vi "Sequencer Main.vi"() -> ()   [LabVIEW 2018] (continued)
                                n1754 = in-place {
                                in-place-border: [w3148] -> w3129
                                in-place-border: w3133 -> [w3147]
                                n1755 = global read "Global Variable.vi" "Rd PID"() -> (w3149:string)
                                n1756 = Equal?(x=w3149, y=w3147) -> (x = y?=w3148:bool)
                                n1757 = global write "Global Variable.vi" "Rd PID RFID"(w3147) -> ()
                                }
                                n1758 = case shown="False" w3129 {
                                tunnel: [w3141 w3142] -> w3131
                                tunnel: w3130 -> [w3140 w3142]
                                frame False {
                                n1759 = Concatenate Strings(w3140, " (False)" ("string")) -> (w3141:string)
                                }
                                frame True {
                                }
                                }
                                n1760 = in-place {
                                in-place-border: w3132 -> [w3144]
                                in-place-border: w3137 -> [w3146]
                                in-place-border: w3138 -> [w3145]
                                in-place-border: [w3143] -> w3135
                                n1761 = In Range and Coerce(upper limit=w3146, x=w3144, lower limit=w3145) -> (In Range?=w3143:bool)  [unwired: 1 out]
                                }
                                n1762 = And(x=w3135, y=w3129) -> (x .and. y?=w3136:bool)
                              }
                            }
                          }
                          n1763 = local read "Debugging"() -> (w3066:bool)
                          n1764 = global read "Global Variable.vi" "Retest Cnt"() -> (w3068:i16)
                          n1765 = in-place {
                            in-place-border: w3070 -> [w3099]
                            in-place-border: [w3098] -> w3069
                            in-place-border: [w3097] -> w3064
                            in-place-border: [w3096] -> w3063
                            # "GoTo Test-nmb"
                            # "ReTest Cyckles"
                            n1766 = Index Array(array=w3099, index #1=0 ("index"), index #2=1 ("index"), index #3=2 ("index")) -> (element #1=w3102:string, element #2=w3101:string, element #3=w3100:string)
                            n1767 = Decimal String To Number(string=w3100) -> (number=w3097:i32)  [unwired: 2 in, 1 out]
                            n1768 = Decimal String To Number(string=w3101) -> (number=w3096:i32)  [unwired: 2 in, 1 out]
                            n1769 = To Upper Case(1:w3102) -> (0:w3098:string)
                          }
                          n1770 = case shown="True" w3074 {
                            tunnel: [enum16{"Idle", "PASS", "FALSE"}."FALSE" ("Step Test Result") enum16{"Idle", "PASS", "FALSE"}."PASS" ("Step Test Result")] -> w3079
                            frame False {
                            }
                            frame True {
                            }
                          }
                          n1771 = Equal?(x=w3068, y=i16 0) -> (x = y?=w3065:bool)
                          n1772 = case shown="False" w3066 {
                            tunnel: w3069 -> [w3083 _]
                            tunnel: w3065 -> [w3080 _]
                            tunnel: w3064 -> [w3082 _]
                            tunnel: w3063 -> [w3081 _]
                            frame False {
                              n1773 = case shown="\"FALSE\"" w3083 {
                                tunnel: w3080 -> [_ w3084]
                                tunnel: w3082 -> [_ w3086]
                                tunnel: w3081 -> [_ w3085]
                                frame "Idle", Default {
                                }
                                frame "FALSE" {
                                n1774 = case shown="False" w3084 {
                                tunnel: w3086 -> [_ w3093]
                                tunnel: w3085 -> [w3088 w3095]
                                frame False {
                                n1775 = global read "Global Variable.vi" "Retest Cnt"() -> (w3091:i16)
                                n1776 = global write "Global Variable.vi" "Retest Step Nmb"(w3088) -> ()
                                n1777 = global write "Global Variable.vi" "Retest ON"(TRUE ("Retest ON")) -> ()
                                n1778 = Decrement(x=w3091) -> (x-1=w3090:i16)
                                n1779 = global write "Global Variable.vi" "Retest Cnt"(w3090) -> ()
                                n1780 = Wait (ms)(milliseconds to wait=u32 1000) -> ()  [unwired: 1 out]
                                }
                                frame True {
                                # "if(Retest-OFF & Cnt=0)"
                                n1781 = Decrement(x=w3093) -> (x-1=w3092:i32)
                                n1782 = global write "Global Variable.vi" "Retest Step Nmb"(w3095) -> ()
                                n1783 = global write "Global Variable.vi" "Retest ON"(TRUE ("Retest ON")) -> ()
                                n1784 = global write "Global Variable.vi" "Retest Cnt"(w3092) -> ()
                                }
                                }
                                }
                              }
                            }
                            frame True {
                            }
                          }
                        }
                        frame 46 {
                          # "GoTo Test-nmb"
                          # "ReTest Cyckles"
                          # "RFID Case\nFTDI"
                          # "Test ADB LMS RFID"
                          n1785 = Unbundle By Name(w3442) -> ("Test Values.Upper Limit"=w3436:dbl, "Test Values.Lower Limit"=w3437:dbl, "Parameters"=w3439:string, "Step Description"=w3428:string)  [unwired: 1 out]
                          n1786 = property on="Tab Control Msg" class="TabCtl (strict)"("Value"=T4."Msg" ("Tab Control Msg")) -> (error out=w3440:errorcluster)  [unwired: 2 in, 1 out]
                          n1787 = in-place {
                            in-place-border: w3440 -> [_]
                            in-place-border: w3439 -> [w3488]
                            in-place-border: [w3482] -> w3438
                            in-place-border: w3437 -> [w3481]
                            in-place-border: w3436 -> [w3480]
                            in-place-border: [w3479] -> w3429
                            in-place-border: [w3477] -> w3435
                            in-place-border: w3428 -> [w3476]
                            in-place-border: [w3476] -> w3427
                            in-place-border: [w3475] -> w3426
                            n1788 = while {
                              shift-right: [w3672] -> _
                              shift-left: w3488 -> [w3673]
                              tunnel: [w3669] -> w3484 mode=indexing
                              stop <- w3671 stop-if-true
                              # "Get Array of Parametrs"
                              n1789 = Match Pattern(string=w3673, regular expression=">") -> (before substring=w3669:string, after substring=w3672:string, offset past match=w3670:i32)  [unwired: 1 in, 1 out]
                              n1790 = Less Than 0?(x=w3670) -> (x < 0?=w3671:bool)
                            }
                            n1791 = Index Array(array=w3484, index #1=0 ("index"), index #2=1 ("index"), index #3=2 ("index")) -> (element #1=w3478:string)  [unwired: 2 out]
                            n1792 = in-place {
                              in-place-border: [w3489] -> w3483
                              # "COMPORT OPEN?"
                              n1793 = global read "Global Variable.vi" "COM Port RFID"() -> (w3491:refnum<visa-resource-name>)
                              n1794 = Not Equal?(x=w3491, y="???") -> (x != y?=w3489:bool)
                            }
                            n1795 = while {
                              shift-right: [w3495] -> _
                              shift-left: w3478 -> [w3496]
                              tunnel: [w3492] -> w3477 mode=indexing
                              stop <- w3494 stop-if-true
                              # "Get Array of Sub Parametrs"
                              n1796 = Match Pattern(string=w3496, regular expression=":") -> (before substring=w3492:string, after substring=w3495:string, offset past match=w3493:i32)  [unwired: 1 in, 1 out]
                              n1797 = Less Or Equal To 0?(x=w3493) -> (x <= 0?=w3494:bool)
                            }
                            n1798 = case shown="True" w3483 {
                              tunnel: [FALSE w3511] -> w3482
                              tunnel: w3481 -> [_ w3513]
                              tunnel: w3480 -> [_ w3512]
                              tunnel: [w3498 w3501] -> w3479
                              tunnel: [w3498 w3500] -> w3475
                              frame False {
                                w3498 = "..."
                              }
                              frame True {
                                n1799 = flat-sequence {
                                tunnel: [w3531] -> w3509
                                tunnel: [w3533] -> w3504
                                tunnel: [w3532] -> w3503
                                tunnel: [w3531] -> w3502
                                tunnel: w3509 -> [w3548]
                                tunnel: [w3553] -> w3506
                                tunnel: [w3539] -> w3508
                                tunnel: [w3547] -> w3507
                                tunnel: w3504 -> [w3549]
                                tunnel: w3503 -> [w3547]
                                tunnel: w3502 -> [w3538]
                                tunnel: [w3538] -> w3500
                                frame #0 {
                                w3526 = "--------------------"
                                w3527 = "\r\n"
                                n1800 = case shown="True" FALSE {
                                frame False {
                                }
                                frame True {
                                n1801 = in-place {
                                # "Debug ONLY!"
                                n1802 = global write "Global Variable.vi" "Rd PID"("2205040012345") -> ()
                                }
                                }
                                }
                                n1803 = Concatenate Strings("Test ADB-LMS FRID", w3527, w3526, w3526, w3527) -> (w3528:string)
                                n1804 = property on="Msg Str" class="Str"("Value"=w3528) -> ()  [unwired: 2 in, 2 out]
                                }
                                frame #1 {
                                n1805 = global read "Global Variable.vi" "COM Port RFID"() -> (w3537:refnum<visa-resource-name>)
                                n1806 = VISA Clear(VISA resource name=w3537) -> (VISA resource name out=w3536:refnum<visa-resource-name>, error out=w3535:errorcluster)  [unwired: 1 in]
                                n1807 = call "RFID_FTDI_Get-ID.vi"("error in"=w3535, "Delay"=u16 1200, "COM RFID"=w3536) -> ("error out"=w3533:errorcluster, "RSSI"=w3532:i32, "Str EPC"=w3531:string)  [unwired: 5 in, 1 out]
                                n1808 = invoke on="Msg Str" class="Str" method="Append String"("string"=w3531) -> ()  [unwired: 3 in, 4 out]
                                }
                                frame #2 {
                                # "RFID PID"
                                n1809 = global read "Global Variable.vi" "Array Errors"() -> (w3552:errorcluster[])
                                n1810 = xnode "Match Regular Expression"("input string"=w3548, "regular expression"="\\[(.*)\\]") -> ("whole match"=w3546:string)  [unwired: 4 in, 4 out]
                                n1811 = Number To Decimal String(number=w3547) -> (decimal integer string=w3543:string)  [unwired: 1 in]
                                n1812 = String Subset(string=w3546, offset (0)=8, length (rest)=13 ("offset (0)")) -> (substring=w3539:string)
                                n1813 = Replace Array Subset(array=w3552, new element=w3549, index=7) -> (w3551:errorcluster[])
                                n1814 = global write "Global Variable.vi" "Array Errors"(w3551) -> ()
                                n1815 = Concatenate Strings(w3543, " (db) ", "\r\n", "                   RFID-PID: " ("string"), w3539) -> (w3553:string)
                                }
                                }
                                n1816 = in-place {
                                in-place-border: [w3524] -> w3505
                                in-place-border: w3508 -> [w3523]
                                n1817 = global read "Global Variable.vi" "Rd PID"() -> (w3522:string)
                                n1818 = global write "Global Variable.vi" "Rd PID RFID"(w3523) -> ()
                                n1819 = Equal?(x=w3522, y=w3523) -> (x = y?=w3524:bool)
                                }
                                n1820 = case shown="True" w3505 {
                                tunnel: [w3516 w3517] -> w3501
                                tunnel: w3506 -> [w3515 w3517]
                                frame False {
                                n1821 = Concatenate Strings(w3515, " (False)" ("string")) -> (w3516:string)
                                }
                                frame True {
                                }
                                }
                                n1822 = in-place {
                                in-place-border: w3507 -> [w3519]
                                in-place-border: w3512 -> [w3521]
                                in-place-border: w3513 -> [w3520]
                                in-place-border: [w3518] -> w3510
                                n1823 = In Range and Coerce(upper limit=w3521, x=w3519, lower limit=w3520) -> (In Range?=w3518:bool)  [unwired: 1 out]
                                }
                                n1824 = And(x=w3510, y=w3505) -> (x .and. y?=w3511:bool)
                              }
                            }
                          }
                          n1825 = local read "Debugging"() -> (w3433:bool)
                          n1826 = in-place {
                            in-place-border: w3435 -> [w3468]
                            in-place-border: [w3467] -> w3434
                            in-place-border: [w3466] -> w3430
                            in-place-border: [w3465] -> w3431
                            n1827 = Index Array(array=w3468, index #1=0 ("index"), index #2=1 ("index"), index #3=2 ("index")) -> (element #1=w3471:string, element #2=w3470:string, element #3=w3469:string)
                            n1828 = Decimal String To Number(string=w3469) -> (number=w3466:i32)  [unwired: 2 in, 1 out]
                            n1829 = Decimal String To Number(string=w3470) -> (number=w3465:i32)  [unwired: 2 in, 1 out]
                            n1830 = To Upper Case(1:w3471) -> (0:w3467:string)
                          }
                          n1831 = in-place {
                            in-place-border: [w3450] -> w3432
                            n1832 = global read "Global Variable.vi" "Retest Cnt"() -> (w3451:i16)
                            n1833 = Equal?(x=w3451, y=i16 0) -> (x = y?=w3450:bool)
                          }
                          n1834 = case shown="False" w3433 {
                            tunnel: w3434 -> [w3455 _]
                            tunnel: w3432 -> [w3452 _]
                            tunnel: w3430 -> [w3454 _]
                            tunnel: w3431 -> [w3453 _]
                            frame False {
                              # "Debug ?"
                              n1835 = case shown="\"FALSE\"" w3455 {
                                tunnel: w3452 -> [_ w3459]
                                tunnel: w3454 -> [_ w3456]
                                tunnel: w3453 -> [_ w3457]
                                frame "Idle", Default {
                                }
                                frame "FALSE" {
                                # "If \"false\" para exixst?"
                                n1836 = global write "Global Variable.vi" "Retest Step Nmb"(w3457) -> ()
                                n1837 = global write "Global Variable.vi" "Retest Nmb"(w3456) -> ()
                                n1838 = case shown="True" w3459 {
                                tunnel: w3456 -> [_ w3464]
                                frame False {
                                # "Else"
                                n1839 = global read "Global Variable.vi" "Retest Cnt"() -> (w3462:i16)
                                n1840 = Decrement(x=w3462) -> (x-1=w3461:i16)
                                n1841 = global write "Global Variable.vi" "Retest Cnt"(w3461) -> ()
                                n1842 = Wait (ms)(milliseconds to wait=u32 1000) -> ()  [unwired: 1 out]
                                }
                                frame True {
                                # "if(Retest-OFF & Cnt=0)"
                                n1843 = Decrement(x=w3464) -> (x-1=w3463:i32)
                                n1844 = global write "Global Variable.vi" "Retest Cnt"(w3463) -> ()
                                }
                                }
                                n1845 = global write "Global Variable.vi" "Retest ON"(TRUE ("Retest ON")) -> ()
                                }
                              }
                            }
                            frame True {
                            }
                          }
                          n1846 = in-place {
                            in-place-border: w3427 -> [w3446]
                            in-place-border: w3426 -> [w3445]
                            in-place-border: w3429 -> [w3444]
                            n1847 = call "Log Add Msg.vi"("Result"=w3444, "Communication"=w3445, "Description"=w3446) -> ("Out Msg"=w3447:string)
                            n1848 = property on="LogMsg" class="Str"("Text.Scroll Position"=inf) -> ()  [unwired: 2 in, 2 out]
                            n1849 = invoke on="LogMsg" class="Str" method="Append String"("string"=w3447) -> ()  [unwired: 3 in, 4 out]
                          }
                          n1850 = case shown="False" w3438 {
                            tunnel: [enum16{"Idle", "PASS", "FALSE"}."FALSE" ("Step Test Result") enum16{"Idle", "PASS", "FALSE"}."PASS" ("Step Test Result")] -> w3443
                            frame False {
                            }
                            frame True {
                            }
                          }
                        }
                        frame 47 {
                          # "FALSE/Idle"
                          # "GoTo Test-nmb"
                          # "ReTest Cyckles"
                          # "RFID Case\nFTDI"
                          # "Test ADB LMS RFID"
                          n1851 = Unbundle By Name(w3693) -> ("Test Values.Upper Limit"=w3687:dbl, "Test Values.Lower Limit"=w3688:dbl, "Parameters"=w3690:string, "Step Description"=w3679:string)  [unwired: 1 out]
                          n1852 = property on="Tab Control Msg" class="TabCtl (strict)"("Value"=T4."Msg" ("Tab Control Msg")) -> (error out=w3691:errorcluster)  [unwired: 2 in, 1 out]
                          n1853 = in-place {
                            in-place-border: w3691 -> [_]
                            in-place-border: w3690 -> [w3739]
                            in-place-border: [w3733] -> w3689
                            in-place-border: w3688 -> [w3732]
                            in-place-border: w3687 -> [w3731]
                            in-place-border: [w3730] -> w3680
                            in-place-border: [w3728] -> w3686
                            in-place-border: w3679 -> [w3727]
                            in-place-border: [w3727] -> w3678
                            in-place-border: [w3726] -> w3677
                            n1854 = while {
                              shift-right: [w3812] -> _
                              shift-left: w3739 -> [w3813]
                              tunnel: [w3809] -> w3735 mode=indexing
                              stop <- w3811 stop-if-true
                              # "Get Array of Parametrs"
                              n1855 = Match Pattern(string=w3813, regular expression=">") -> (before substring=w3809:string, after substring=w3812:string, offset past match=w3810:i32)  [unwired: 1 in, 1 out]
                              n1856 = Less Than 0?(x=w3810) -> (x < 0?=w3811:bool)
                            }
                            n1857 = Index Array(array=w3735, index #1=0 ("index"), index #2=1 ("index"), index #3=2 ("index")) -> (element #1=w3729:string)  [unwired: 2 out]
                            n1858 = in-place {
                              in-place-border: [w3740] -> w3734
                              # "COMPORT OPEN?"
                              n1859 = global read "Global Variable.vi" "COM Port RFID"() -> (w3742:refnum<visa-resource-name>)
                              n1860 = Not Equal?(x=w3742, y="???") -> (x != y?=w3740:bool)
                            }
                            n1861 = while {
                              shift-right: [w3746] -> _
                              shift-left: w3729 -> [w3747]
                              tunnel: [w3743] -> w3728 mode=indexing
                              stop <- w3745 stop-if-true
                              # "Get Array of Sub Parametrs"
                              n1862 = Match Pattern(string=w3747, regular expression=":") -> (before substring=w3743:string, after substring=w3746:string, offset past match=w3744:i32)  [unwired: 1 in, 1 out]
                              n1863 = Less Or Equal To 0?(x=w3744) -> (x <= 0?=w3745:bool)
                            }
                            n1864 = case shown="True" w3734 {
                              tunnel: [FALSE w3765] -> w3733
                              tunnel: w3732 -> [_ w3767]
                              tunnel: w3731 -> [_ w3766]
                              tunnel: [w3749 w3756] -> w3730
                              tunnel: [w3749 w3755] -> w3726
                              frame False {
                                w3749 = "..."
                              }
                              frame True {
                                n1865 = flat-sequence {
                                tunnel: [w3779] -> w3752
                                tunnel: w3752 -> [w3787]
                                tunnel: [w3787] -> w3751
                                tunnel: [w3790] -> w3759
                                tunnel: [w3791] -> w3758
                                tunnel: [w3789] -> w3757
                                tunnel: [w3789] -> w3754
                                tunnel: w3751 -> [w3788]
                                tunnel: [w3808] -> w3761
                                tunnel: [w3799] -> w3763
                                tunnel: [w3798] -> w3762
                                tunnel: w3759 -> [w3804]
                                tunnel: w3758 -> [w3798]
                                tunnel: w3757 -> [w3797]
                                tunnel: [w3797] -> w3755
                                tunnel: w3754 -> [w3801]
                                tunnel: [w3795] -> w3753
                                frame #0 {
                                w3781 = "--------------------"
                                w3782 = "\r\n"
                                n1866 = global read "Global Variable.vi" "COM Port RFID"() -> (w3779:refnum<visa-resource-name>)
                                n1867 = case shown="True" FALSE {
                                frame False {
                                }
                                frame True {
                                n1868 = in-place {
                                # "Debug ONLY!"
                                n1869 = global write "Global Variable.vi" "Rd PID"("2205040012345") -> ()
                                }
                                }
                                }
                                n1870 = Concatenate Strings("Test ADB-LMS FRID M5", w3782, w3781, w3781, w3782) -> (w3783:string)
                                n1871 = property on="Msg Str" class="Str"("Value"=w3783) -> ()  [unwired: 2 in, 2 out]
                                }
                                frame #1 {
                                n1872 = call "setTxPower.vi"("db"=u16 100, "ComPort"=w3787) -> ()  [unwired: 8 in, 2 out]
                                }
                                frame #2 {
                                n1873 = call "pollingOnce.vi"("Rd Deelay"=u16 250 ("Delay"), "ComPort"=w3788) -> ("error out"=w3790:errorcluster, "rssi"=w3791:i16, "LMS: PID"=w3789:string)  [unwired: 6 in, 1 out]
                                }
                                frame #3 {
                                w3793 = " (db) "
                                # "RFID PID"
                                n1874 = global read "Global Variable.vi" "Array Errors"() -> (w3807:errorcluster[])
                                n1875 = Number To Decimal String(number=w3798) -> (decimal integer string=w3794:string)  [unwired: 1 in]
                                n1876 = Match Pattern(string=w3801, regular expression="LED-LMS") -> (after substring=w3799:string)  [unwired: 1 in, 3 out]
                                n1877 = Replace Array Subset(array=w3807, new element=w3804, index=7) -> (w3806:errorcluster[])
                                n1878 = global write "Global Variable.vi" "Array Errors"(w3806) -> ()
                                n1879 = Concatenate Strings(w3794, w3793, "\r", "                   RFID-PID: " ("string"), w3799) -> (w3808:string)
                                n1880 = Concatenate Strings(w3797, " : ", w3794, w3793) -> (w3795:string)
                                }
                                }
                                n1881 = invoke on="Msg Str" class="Str" method="Append String"("string"=w3753) -> ()  [unwired: 3 in, 4 out]
                                n1882 = in-place {
                                in-place-border: [w3778] -> w3760
                                in-place-border: w3763 -> [w3777]
                                n1883 = global read "Global Variable.vi" "Baccode MEM"() -> (w3776:string)
                                n1884 = global write "Global Variable.vi" "Rd PID RFID"(w3777) -> ()
                                n1885 = Equal?(x=w3776, y=w3777) -> (x = y?=w3778:bool)
                                }
                                n1886 = case shown="False" w3760 {
                                tunnel: [w3770 w3771] -> w3756
                                tunnel: w3761 -> [w3769 w3771]
                                frame False {
                                n1887 = Concatenate Strings(w3769, " (False)" ("string")) -> (w3770:string)
                                }
                                frame True {
                                }
                                }
                                n1888 = in-place {
                                in-place-border: w3762 -> [w3773]
                                in-place-border: w3766 -> [w3775]
                                in-place-border: w3767 -> [w3774]
                                in-place-border: [w3772] -> w3764
                                n1889 = In Range and Coerce(upper limit=w3775, x=w3773, lower limit=w3774) -> (In Range?=w3772:bool)  [unwired: 1 out]
                                }
                                n1890 = And(x=w3764, y=w3760) -> (x .and. y?=w3765:bool)
                              }
                            }
                          }
                          n1891 = local read "Debugging"() -> (w3684:bool)
                          n1892 = in-place {
                            in-place-border: w3686 -> [w3719]
                            in-place-border: [w3718] -> w3685
                            in-place-border: [w3717] -> w3681
                            in-place-border: [w3716] -> w3682
                            # "Retest Parameters"
                            n1893 = Index Array(array=w3719, index #1=0 ("index"), index #2=1 ("index"), index #3=2 ("index")) -> (element #1=w3722:string, element #2=w3721:string, element #3=w3720:string)
                            n1894 = Decimal String To Number(string=w3720) -> (number=w3717:i32)  [unwired: 2 in, 1 out]
                            n1895 = Decimal String To Number(string=w3721) -> (number=w3716:i32)  [unwired: 2 in, 1 out]
                            n1896 = To Upper Case(1:w3722) -> (0:w3718:string)
                          }
                          n1897 = in-place {
                            in-place-border: [w3701] -> w3683
                            n1898 = global read "Global Variable.vi" "Retest Cnt"() -> (w3702:i16)
                            n1899 = Equal?(x=w3702, y=i16 0) -> (x = y?=w3701:bool)
                          }
                          n1900 = case shown="False" w3684 {
                            tunnel: w3685 -> [w3706 _]
                            tunnel: w3683 -> [w3703 _]
                            tunnel: w3681 -> [w3705 _]
                            tunnel: w3682 -> [w3704 _]
                            frame False {
                              # "Debug ?"
                              n1901 = case shown="\"FALSE\"" w3706 {
                                tunnel: w3703 -> [_ w3710]
                                tunnel: w3705 -> [_ w3707]
                                tunnel: w3704 -> [_ w3708]
                                frame "Idle", Default {
                                }
                                frame "FALSE" {
                                # "If \"false\" para exixst?"
                                n1902 = global write "Global Variable.vi" "Retest Step Nmb"(w3708) -> ()
                                n1903 = global write "Global Variable.vi" "Retest Nmb"(w3707) -> ()
                                n1904 = case shown="True" w3710 {
                                tunnel: w3707 -> [_ w3715]
                                frame False {
                                # "Else"
                                n1905 = global read "Global Variable.vi" "Retest Cnt"() -> (w3713:i16)
                                n1906 = Decrement(x=w3713) -> (x-1=w3712:i16)
                                n1907 = global write "Global Variable.vi" "Retest Cnt"(w3712) -> ()
                                n1908 = Wait (ms)(milliseconds to wait=u32 1000) -> ()  [unwired: 1 out]
                                }
                                frame True {
                                # "if(Retest-OFF & Cnt=0)"
                                n1909 = Decrement(x=w3715) -> (x-1=w3714:i32)
                                n1910 = global write "Global Variable.vi" "Retest Cnt"(w3714) -> ()
                                }
                                }
                                n1911 = global write "Global Variable.vi" "Retest ON"(TRUE ("Retest ON")) -> ()
                                }
                              }
                            }
                            frame True {
                            }
                          }
                          n1912 = in-place {
                            in-place-border: w3678 -> [w3697]
                            in-place-border: w3677 -> [w3696]
                            in-place-border: w3680 -> [w3695]
                            n1913 = call "Log Add Msg.vi"("Result"=w3695, "Communication"=w3696, "Description"=w3697) -> ("Out Msg"=w3698:string)
                            n1914 = property on="LogMsg" class="Str"("Text.Scroll Position"=inf) -> ()  [unwired: 2 in, 2 out]
                            n1915 = invoke on="LogMsg" class="Str" method="Append String"("string"=w3698) -> ()  [unwired: 3 in, 4 out]
                          }
                          n1916 = case shown="False" w3689 {
                            tunnel: [enum16{"Idle", "PASS", "FALSE"}."FALSE" ("Step Test Result") enum16{"Idle", "PASS", "FALSE"}."PASS" ("Step Test Result")] -> w3694
                            frame False {
                            }
                            frame True {
                            }
                          }
                        }
                        frame 50 {
                          # "Lover Lim"
                          # "Upper Lim"
                          # "PicoScope\n Case"
                          # "PicoScope Case"
                          n1917 = Unbundle By Name(w3833) -> ("Test Values.Upper Limit"=w3831:dbl, "Test Values.Lower Limit"=w3830:dbl, "Test Values.Numeric Value"=w3832:dbl)  [unwired: 1 out]
                          n1918 = property on="Tab Control Msg" class="TabCtl (strict)"("Value"=T21."Scope" ("Tab Control Msg")) -> (error out=w3829:errorcluster)  [unwired: 2 in, 1 out]
                          n1919 = flat-sequence {
                            tunnel: w3832 -> [w3866]
                            tunnel: w3831 -> [w3857]
                            tunnel: w3830 -> [w3856]
                            tunnel: w3829 -> [_]
                            tunnel: [w3857] -> w3820
                            tunnel: [w3856] -> w3819
                            tunnel: [w3870] -> w3828
                            tunnel: w3828 -> [w3894]
                            tunnel: [w3894] -> w3823
                            tunnel: [w3882] -> w3822
                            tunnel: [w3881] -> w3821
                            frame #0 {
                              n1920 = control-ref of="Channel B"() -> (w3859:refnum<vi>)
                              n1921 = control-ref of="Channel A"() -> (w3860:refnum<vi>)
                              n1922 = Multiply(x=w3856, y=-0.2) -> (x*y=w3861:dbl)
                              n1923 = Bundle("Lower Limit"=w3856, "Upper Limit"=w3857, "Numeric Value"=w3866) -> (w3867:T36)  [unwired: 1 in]
                              n1924 = Multiply(x=w3857, y=0.2) -> (x*y=w3863:dbl)
                              n1925 = Add(x=w3861, y=w3856) -> (x+y=w3858:dbl)
                              n1926 = property on="Limits" class="Slide (strict)"("Value"=w3867) -> ()  [unwired: 2 in, 2 out]
                              n1927 = invoke class="WFGraph (strict)" method="Reinit To Default"(reference=w3860) -> ()  [unwired: 2 in, 3 out]
                              n1928 = invoke class="WFGraph (strict)" method="Reinit To Default"(reference=w3859) -> ()  [unwired: 2 in, 3 out]
                              n1929 = Add(x=w3863, y=w3857) -> (x+y=w3862:dbl)
                              n1930 = property on="Limits" class="Slide (strict)"("Scale.Maximum"=w3862, "Scale.Minimum"=w3858) -> ()  [unwired: 2 in, 2 out]
                            }
                            frame #1 {
                              # "Ch B"
                              # "Ch A"
                              # "Trigger"
                              # "Err From PicoScope"
                              # "Read PicoScope"
                              n1931 = global read "Global Variable.vi" "Array Errors"() -> (w3880:errorcluster[])
                              n1932 = global read "Global Variable.vi" "PicoScope Max Adc Value"() -> (w3873:i16)
                              n1933 = global read "Global Variable.vi" "PicoScope Device Info"() -> (w3877:T35)
                              n1934 = global read "Global Variable.vi" "PicoScope Handle"() -> (w3878:u32)
                              n1935 = Index Array(array=w3880, index=5) -> (element=w3872:errorcluster)
                              n1936 = control-ref of="Channel A"() -> (w3869:refnum<vi>)
                              n1937 = control-ref of="Channel B"() -> (w3868:refnum<vi>)
                              n1938 = call "PicoScope-3000 Read.vi"("WFD-Ref Ch-B"=w3868, "WFD-Ref Ch-A"=w3869, "Acquisition Settings"=T26 {"preTriggerSamples"=0, "postTriggerSamples"=1000, "timebase"=62500, "Down-Sample Mode"=0, "Down Sample Ratio"=1}, "Trigger Settings"=T28 {"Trigger Enabled"=TRUE, "Trigger Source"=enum."Channel A", "Trigger Threshold (Volts)"=0.0, "Trigger Direction"=2, "Trigger Delay (samples)"=0, "Auto Trigger Time (ms)"=2000}, "Channel B Settings"=T27 {"Enabled"=TRUE, "Coupling"=0, "Range"=10, "Analogue Offset"=0.0}, "Channel A Settings"=T27 {"Enabled"=TRUE, "Coupling"=0, "Range"=10, "Analogue Offset"=0.0}, "error in"=w3872, "Max Adc value"=w3873, "Device Info"=w3877, "handle"=w3878) -> ("error out"=w3870:errorcluster)  [unwired: 1 out]
                            }
                            frame #2 {
                              w3883 = 11.25
                              # "Negative Vmin"
                              # "Positive Vmax"
                              # "Res Devider Compens\n100K / 10K"
                              # "Calculate Values"
                              n1939 = local read "Channel A"() -> (w3908:cluster{i32, dbl, dbl[]})
                              n1940 = local read "Channel B"() -> (w3901:cluster{i32, dbl, dbl[]})
                              n1941 = Unbundle(w3908) -> (w3905:dbl[])  [unwired: 2 out]
                              n1942 = Unbundle(w3901) -> (w3897:dbl[])  [unwired: 2 out]
                              n1943 = call-poly <vilib>:"Basic Averaged DC-RMS.vi"("signal in"=w3905) -> ("RMS value"=w3893:dbl, "DC value"=w3902:dbl)  [unwired: 7 in, 2 out]
                              n1944 = Array Max & Min(array=w3905) -> (max value=w3904:dbl, min value=w3903:dbl)  [unwired: 2 out]
                              n1945 = call-poly <vilib>:"Basic Averaged DC-RMS.vi"("signal in"=w3897) -> ("RMS value"=w3889:dbl, "DC value"=w3900:dbl)  [unwired: 7 in, 2 out]
                              n1946 = Array Max & Min(array=w3897) -> (max value=w3898:dbl, min value=w3899:dbl)  [unwired: 2 out]
                              n1947 = Subtract(x=w3904, y=w3902) -> (x-y=w3892:dbl)
                              n1948 = Add(x=w3903, y=w3902) -> (x+y=w3891:dbl)
                              n1949 = Subtract(x=w3898, y=w3900) -> (x-y=w3887:dbl)
                              n1950 = Add(x=w3899, y=w3900) -> (x+y=w3886:dbl)
                              n1951 = Multiply(x=w3893, y=w3883) -> (x*y=w3890:dbl)
                              n1952 = Multiply(x=w3892, y=w3883) -> (x*y=w3882:dbl)
                              n1953 = Multiply(x=w3891, y=w3883) -> (x*y=w3881:dbl)
                              n1954 = local read "Measure Ch-A"() -> (w3907:T10)
                              n1955 = Multiply(x=w3889, y=w3883) -> (x*y=w3888:dbl)
                              n1956 = Multiply(x=w3887, y=w3883) -> (x*y=w3885:dbl)
                              n1957 = Multiply(x=w3886, y=w3883) -> (x*y=w3884:dbl)
                              n1958 = local read "Measure Ch-B"() -> (w3895:T9)
                              n1959 = Bundle By Name(cluster=w3907, "MAX Vpp"=w3882, "PickToPoick / 2"=w3890, "MIN Vpp"=w3881) -> (w3906:T10)
                              n1960 = local write "Measure Ch-A"(w3906) -> ()
                              n1961 = Bundle By Name(cluster=w3895, "MAX Vpp"=w3885, "PickToPick / 2"=w3888, "MIN Vpp"=w3884) -> (w3896:T9)
                              n1962 = local write "Measure Ch-B"(w3896) -> ()
                            }
                          }
                          n1963 = global read "Global Variable.vi" "Array Errors"() -> (w3825:errorcluster[])
                          n1964 = Replace Array Subset(array=w3825, new element=w3823, index=5) -> (w3826:errorcluster[])
                          n1965 = in-place {
                            in-place-border: w3822 -> [w3837]
                            in-place-border: w3821 -> [w3836]
                            in-place-border: w3820 -> [w3846]
                            in-place-border: w3819 -> [w3845]
                            in-place-border: [w3847] -> w3818
                            in-place-border: [w3835] -> w3817
                            # "Step TEST Result"
                            n1966 = in-place {
                              in-place-border: w3846 -> [w3851]
                              in-place-border: w3845 -> [w3848]
                              in-place-border: [w3851] -> w3844
                              in-place-border: [w3850] -> w3842
                              in-place-border: [w3849] -> w3841
                              in-place-border: [w3848] -> w3843
                              n1967 = Multiply(x=w3848, y=-1.0) -> (x*y=w3849:dbl)
                              n1968 = Multiply(x=w3851, y=-1.0) -> (x*y=w3850:dbl)
                            }
                            n1969 = In Range and Coerce(upper limit=w3844, x=w3837, lower limit=w3843) -> (In Range?=w3840:bool)  [unwired: 1 out]
                            n1970 = In Range and Coerce(upper limit=w3841, x=w3836, lower limit=w3842) -> (In Range?=w3839:bool)  [unwired: 1 out]
                            n1971 = And(x=w3840, y=w3839) -> (x .and. y?=w3838:bool)
                            n1972 = Format Into String(format string="Max: %.1fVAC :: Min: %.1fVAC", w3837, w3836) -> (resulting string=w3835:string)  [unwired: 2 in, 1 out]
                            n1973 = case shown="False" w3838 {
                              tunnel: [enum16{"Idle", "PASS", "FALSE"}."FALSE" ("Step Test Result") enum16{"Idle", "PASS", "FALSE"}."PASS" ("Step Test Result")] -> w3847
                              frame False {
                              }
                              frame True {
                              }
                            }
                          }
                          n1974 = global write "Global Variable.vi" "Array Errors"(w3826) -> ()
                        }
                        frame 51 {
                          # "Create Thread Asynchronous"
                          # "PicoScope\n Case"
                          # "PicoScope Case"
                          n1975 = Unbundle By Name(w3925) -> ("Parameters"=w3912:string, "Test Values.Upper Limit"=w3923:dbl, "Test Values.Lower Limit"=w3922:dbl, "Test Values.Numeric Value"=w3924:dbl, "Step Description"=w3910:string)
                          n1976 = property on="Tab Control Msg" class="TabCtl (strict)"("Value"=T21."Msg" ("Tab Control Msg")) -> (error out=w3921:errorcluster)  [unwired: 2 in, 1 out]
                          n1977 = flat-sequence {
                            tunnel: w3924 -> [w3941]
                            tunnel: w3923 -> [w3932]
                            tunnel: w3922 -> [w3931]
                            tunnel: w3921 -> [_]
                            tunnel: [w3932] -> _
                            tunnel: [w3931] -> _
                            tunnel: w3912 -> [w3930]
                            tunnel: [w3929] -> w3911
                            tunnel: w3910 -> [w3928]
                            tunnel: [w3928] -> w3909
                            tunnel: [w3984] -> w3915
                            tunnel: w3911 -> [w3974]
                            tunnel: w3909 -> [w3961]
                            frame #0 {
                              n1978 = control-ref of="Channel B"() -> (w3934:refnum<vi>)
                              n1979 = control-ref of="Channel A"() -> (w3935:refnum<vi>)
                              n1980 = Multiply(x=w3931, y=-0.2) -> (x*y=w3936:dbl)
                              n1981 = Bundle("Lower Limit"=w3931, "Upper Limit"=w3932, "Numeric Value"=w3941) -> (w3942:T36)  [unwired: 1 in]
                              n1982 = while {
                                shift-right: [w3946] -> _
                                shift-left: w3930 -> [w3947]
                                tunnel: [w3943] -> w3929 mode=indexing
                                stop <- w3945 stop-if-true
                                # "Get Array of Parametrs"
                                n1983 = Match Pattern(string=w3947, regular expression=">") -> (before substring=w3943:string, after substring=w3946:string, offset past match=w3944:i32)  [unwired: 1 in, 1 out]
                                n1984 = Less Than 0?(x=w3944) -> (x < 0?=w3945:bool)
                              }
                              n1985 = Multiply(x=w3932, y=0.2) -> (x*y=w3938:dbl)
                              n1986 = Add(x=w3936, y=w3931) -> (x+y=w3933:dbl)
                              n1987 = property on="Limits" class="Slide (strict)"("Value"=w3942) -> ()  [unwired: 2 in, 2 out]
                              n1988 = Add(x=w3938, y=w3932) -> (x+y=w3937:dbl)
                              n1989 = invoke class="WFGraph (strict)" method="Reinit To Default"(reference=w3935) -> ()  [unwired: 2 in, 3 out]
                              n1990 = invoke class="WFGraph (strict)" method="Reinit To Default"(reference=w3934) -> ()  [unwired: 2 in, 3 out]
                              n1991 = property on="Limits" class="Slide (strict)"("Scale.Maximum"=w3937, "Scale.Minimum"=w3933) -> ()  [unwired: 2 in, 2 out]
                            }
                            frame #1 {
                              w3959 = "----------------------"
                              w3960 = "\r\n"
                              # "Ch B"
                              # "Ch A"
                              # "Trigger"
                              # "Read PicoScope"
                              n1992 = vi-ref "PicoScope-3000 Read.vi"() -> (w3953:refnum<vi>)
                              n1993 = Index Array(array=w3974, index #1=0 ("index"), index #2=1 ("index"), index #3=2 ("index")) -> (element #1=w3970:string, element #2=w3966:string, element #3=w3964:string)
                              n1994 = property class="VI"(reference=w3953) -> (error out=w3955:errorcluster, "Path"=w3957:path)  [unwired: 1 in, 1 out]
                              n1995 = Decimal String To Number(string=w3966) -> (number=w3969:i32)  [unwired: 2 in, 1 out]
                              n1996 = Decimal String To Number(string=w3964) -> (number=w3968:i32)  [unwired: 2 in, 1 out]
                              n1997 = global read "Global Variable.vi" "PicoScope Max Adc Value"() -> (w3979:i16)
                              n1998 = case shown="\"A\", Default" w3970 {
                                tunnel: [T28 {"Trigger Enabled"=TRUE, "Trigger Source"=enum."Channel A", "Trigger Threshold (Volts)"=0.1, "Trigger Direction"=2, "Trigger Delay (samples)"=0, "Auto Trigger Time (ms)"=2000} ("Trigger Settings") T28 {"Trigger Enabled"=TRUE, "Trigger Source"=enum."Channel B", "Trigger Threshold (Volts)"=0.1, "Trigger Direction"=2, "Trigger Delay (samples)"=0, "Auto Trigger Time (ms)"=3000} ("Trigger Settings")] -> w3958
                                tunnel: ["Trig: Ch-A" "Trig: Ch-B"] -> w3962
                                frame "A", Default {
                                }
                                frame "B" {
                                }
                              }
                              n1999 = global read "Global Variable.vi" "PicoScope Device Info"() -> (w3980:T35)
                              n2000 = global read "Global Variable.vi" "PicoScope Handle"() -> (w3981:u32)
                              n2001 = Open VI Reference(type specifier VI Refnum (for type only)=refnum<vi> refnum, vi path=w3957, options=128, error in (no error)=w3955) -> (vi reference=w3949:refnum<vi>, error out=w3983:errorcluster)  [unwired: 2 in]
                              n2002 = Bundle By Name(cluster=T26 {"preTriggerSamples"=0, "postTriggerSamples"=10000, "timebase"=5000, "Down-Sample Mode"=0, "Down Sample Ratio"=1} ("Acquisition Settings"), "postTriggerSamples"=w3969, "timebase"=w3968) -> (w3951:T26)
                              n2003 = control-ref of="Channel A"() -> (w3975:refnum<vi>)
                              n2004 = control-ref of="Channel B"() -> (w3977:refnum<vi>)
                              n2005 = call-by-ref "Start Asynchronous Call"(reference=w3949, error in=w3983, "WFD-Ref Ch-B"=w3977, "WFD-Ref Ch-A"=w3975, "Acquisition Settings"=w3951, "Trigger Settings"=w3958, "Channel B Settings"=T27 {"Enabled"=TRUE, "Coupling"=0, "Range"=6, "Analogue Offset"=0.0}, "Channel A Settings"=T27 {"Enabled"=TRUE, "Coupling"=0, "Range"=6, "Analogue Offset"=0.0}, "Max Adc value"=w3979, "Device Info"=w3980, "handle"=w3981) -> (reference out=w3976:refnum<vi>, error out=w3954:errorcluster)  [unwired: 1 in, 2 out]
                              n2006 = case shown="Error" w3954 {
                                frame No Error {
                                }
                                frame Error {
                                n2007 = One Button Dialog(message="PycoScope Err") -> ()  [unwired: 1 in, 1 out]
                                }
                              }
                              n2008 = Concatenate Strings(w3961, w3960, w3959, w3959, w3960, w3962, w3960, "Samples: ", w3966, w3960, "Base Time: ", w3964, w3960) -> (w3963:string)
                              n2009 = Close Reference(reference=w3976, error in (no error)=w3954) -> (error out=w3984:errorcluster)
                              n2010 = local write "Msg Str"(w3963) -> ()
                            }
                          }
                          n2011 = global read "Global Variable.vi" "Array Errors"() -> (w3918:errorcluster[])
                          n2012 = Replace Array Subset(array=w3918, new element=w3915, index=5) -> (w3919:errorcluster[])
                          n2013 = global write "Global Variable.vi" "Array Errors"(w3919) -> ()
                          n2014 = Unbundle By Name(w3915) -> ("status"=w3914:bool)
                          n2015 = Not(x=w3914) -> (.not. x?=w3913:bool)
                          n2016 = case shown="True" w3913 {
                            tunnel: [enum16{"Idle", "PASS", "FALSE"}."FALSE" ("Step Test Result") enum16{"Idle", "PASS", "FALSE"}."Idle" ("Step Test Result")] -> w3916
                            frame False {
                            }
                            frame True {
                            }
                          }
                        }
                        frame 52 {
                          # "Read Positive & negative Values"
                          # "Lover Lim"
                          # "Upper Lim"
                          # "PicoScope\n Case"
                          # "PicoScope Case"
                          n2017 = Unbundle By Name(w4012) -> ("Parameters"=w4006:string, "Test Values.Upper Limit"=w4010:dbl, "Test Values.Lower Limit"=w4009:dbl, "Test Values.Numeric Value"=w4011:dbl)
                          n2018 = property on="Tab Control Msg" class="TabCtl (strict)"("Value"=T21."Scope" ("Tab Control Msg")) -> (error out=w4008:errorcluster)  [unwired: 2 in, 1 out]
                          n2019 = flat-sequence {
                            tunnel: w4011 -> [w4050]
                            tunnel: w4010 -> [w4043]
                            tunnel: w4009 -> [w4042]
                            tunnel: w4008 -> [_]
                            tunnel: [w4043] -> w3996
                            tunnel: [w4042] -> w3997
                            tunnel: w4006 -> [w4041]
                            tunnel: [w4039] -> w4001
                            tunnel: [w4035] -> w3998
                            tunnel: [w4103] -> w4005
                            tunnel: [w4102] -> w4004
                            tunnel: [w4101] -> w4003
                            tunnel: [w4100] -> w4002
                            tunnel: w4001 -> [w4092]
                            tunnel: [w4092] -> w4000
                            tunnel: [w4091] -> w3999
                            tunnel: w3998 -> [w4091]
                            tunnel: w4005 -> [w4123]
                            tunnel: w4004 -> [w4122]
                            tunnel: w4003 -> [w4121]
                            tunnel: w4002 -> [w4120]
                            tunnel: w4000 -> [w4138]
                            tunnel: w3999 -> [w4131]
                            tunnel: [w4115] -> w3994
                            tunnel: [w4114] -> w3992
                            tunnel: [w4156] -> w3995
                            tunnel: w3994 -> [w4156]
                            tunnel: [w4155] -> w3993
                            tunnel: w3992 -> [w4155]
                            frame #0 {
                              n2020 = while {
                                shift-right: [w4061] -> _
                                shift-left: w4041 -> [w4062]
                                tunnel: [w4058] -> w4040 mode=indexing
                                stop <- w4060 stop-if-true
                                # "Get Array of Parametrs"
                                n2021 = Match Pattern(string=w4062, regular expression=">") -> (before substring=w4058:string, after substring=w4061:string, offset past match=w4059:i32)  [unwired: 1 in, 1 out]
                                n2022 = Less Than 0?(x=w4059) -> (x < 0?=w4060:bool)
                              }
                              n2023 = Multiply(x=w4042, y=-0.2) -> (x*y=w4045:dbl)
                              n2024 = Bundle("Lower Limit"=w4042, "Upper Limit"=w4043, "Numeric Value"=w4050) -> (w4051:T36)  [unwired: 1 in]
                              n2025 = Multiply(x=w4043, y=0.2) -> (x*y=w4047:dbl)
                              n2026 = Add(x=w4045, y=w4042) -> (x+y=w4044:dbl)
                              n2027 = property on="Limits" class="Slide (strict)"("Value"=w4051) -> ()  [unwired: 2 in, 2 out]
                              n2028 = Add(x=w4047, y=w4043) -> (x+y=w4046:dbl)
                              n2029 = property on="Limits" class="Slide (strict)"("Scale.Maximum"=w4046, "Scale.Minimum"=w4044) -> ()  [unwired: 2 in, 2 out]
                              n2030 = Index Array(array=w4040, index #1=0 ("index"), index #2=1 ("index")) -> (element #1=w4039:string, element #2=w4036:string)
                              n2031 = while {
                                shift-right: [w4055] -> _
                                shift-left: w4036 -> [w4056]
                                tunnel: [w4052] -> w4035 mode=indexing
                                stop <- w4054 stop-if-true
                                # "Get Array of Sub Parametrs"
                                n2032 = Match Pattern(string=w4056, regular expression=":") -> (before substring=w4052:string, after substring=w4055:string, offset past match=w4053:i32)  [unwired: 1 in, 1 out]
                                n2033 = Less Than 0?(x=w4053) -> (x < 0?=w4054:bool)
                              }
                            }
                            frame #1 {
                              w4064 = TRUE
                              w4095 = 100 ("index")
                              # "700"
                              # "302"
                              # "Devider compensite"
                              # "remove first\nxx element (noise)"
                              # "Ch-B Negative Vmin"
                              # "Ch-B Positive Vmax"
                              # "Ch-A Negative Vmin"
                              # "Ch-A Positive Vmax"
                              # "Res Devider Compens\n100K / 10K"
